vi "NoneScript.vi"(11 "base path":path) -> ()   [LabVIEW 2019, in "Scripts.lvclass"]
uses:
  Scripts.lvclass
  <vilib>/Utility/file.llb/Write Delimited Spreadsheet (string).vi
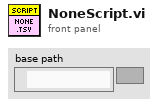
[diagram p1: front panel]
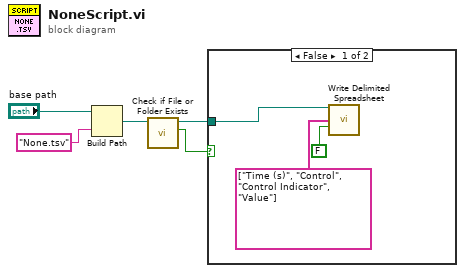
[diagram p0: block diagram]
diagram:
  n1 = Build Path(base path="base path", name or relative path="None.tsv") -> (appended path=w4:path)
  n2 = call <vilib>:"Check if File or Folder Exists.vi"("path"=w4) -> ("file or folder exists?"=w3:bool, "dup path"=w2:path)  [unwired: 8 in, 1 out]
  n3 = case shown="False" w3 {
    tunnel: w2 -> [w7 _]
    frame False {
      n4 = call-poly <vilib>:"Write Delimited Spreadsheet.vi"("file path (dialog if empty)"=w7, "1D data"=string[] ["Time (s)", "Control", "Control Indicator", "Value"], "append to file? (new file:F)"=FALSE) -> ()  [unwired: 11 in, 2 out]
    }
    frame True {
    }
  }
